vi "Region-det-diagnostics.vi"() -> ()   [LabVIEW 2016]
panel:
  out "Region 3":dbl
  out "millisec gen Q mat":u32
  out "millisec det reg":u32
  out "Region 2":dbl
  out "Region":dbl
  in  "State":dbl[](array[numeric])
  out "Q Matrices":dbl[][][][](array[numeric])
  # "Just for diagnostics (to record the amount of time it takes to load a JSON file as compared with the amount of time to determine the region"
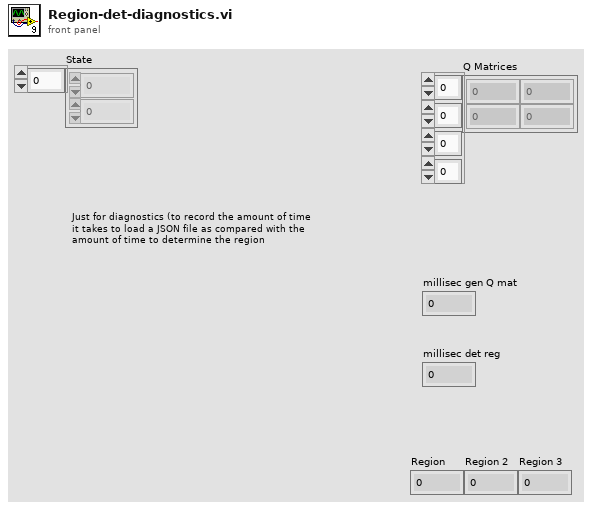
[diagram p1: front panel]
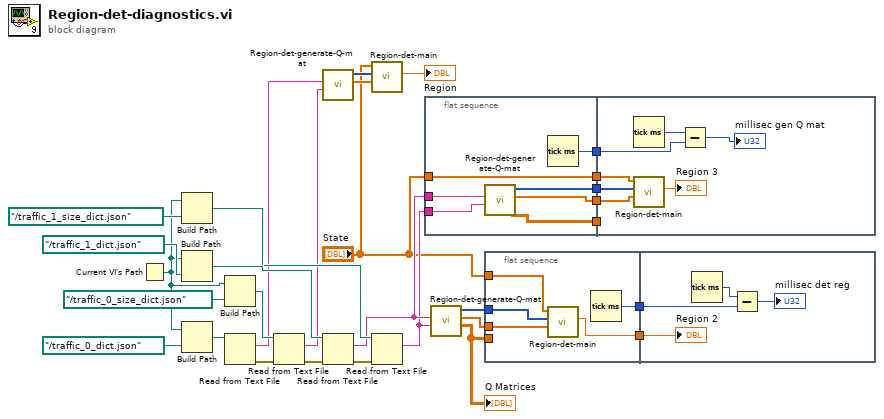
[diagram p0: block diagram]
diagram:
  n1 = Current VI's Path() -> (path=w22:path)
  n2 = Build Path(base path=w22, name or relative path=path "../traffic_1_size_dict.json") -> (appended path=w23:path)
  n3 = Build Path(base path=w22, name or relative path=path "../traffic_1_dict.json") -> (appended path=w26:path)
  n4 = Build Path(base path=w22, name or relative path=path "../traffic_0_dict.json") -> (appended path=w30:path)
  n5 = Build Path(base path=w22, name or relative path=path "../traffic_0_size_dict.json") -> (appended path=w27:path)
  n6 = Read from Text File(file (use dialog)=w30) -> (text=w18:string, error out=w21:errorcluster)  [unwired: 3 in, 2 out]
  n7 = Read from Text File(file (use dialog)=w27, error in=w21) -> (text=w17:string, error out=w20:errorcluster)  [unwired: 2 in, 2 out]
  n8 = call "Region-det-generate-Q-mat.vi"("Q region size JSON string"=w17, "Q matrix JSON string"=w18) -> ("Index array"=w14:dbl[], "Regions"=w16:i32[])  [unwired: 6 in, 2 out]
  n9 = Read from Text File(file (use dialog)=w26, error in=w20) -> (text=w7:string, error out=w19:errorcluster)  [unwired: 2 in, 2 out]
  n10 = call "Region-det-main.vi"("Index Array"=w14, "Regions"=w16, "State"="State") -> ("Region"=→"Region":dbl)  [unwired: 8 in]
  n11 = Read from Text File(file (use dialog)=w23, error in=w19) -> (text=w6:string)  [unwired: 2 in, 3 out]
  n12 = flat-sequence {
    tunnel: [w37] -> w8
    tunnel: w7 -> [w36]
    tunnel: w6 -> [w35]
    tunnel: [w34] -> w5
    tunnel: "State" -> [w33]
    tunnel: [w33] -> w3
    tunnel: [w32] -> w2
    tunnel: [w31] -> w1
    tunnel: w8 -> [w43]
    tunnel: w5 -> [_]
    tunnel: w3 -> [w41]
    tunnel: w2 -> [w40]
    tunnel: w1 -> [w39]
    frame #0 {
      n13 = call "Region-det-generate-Q-mat.vi"("Q region size JSON string"=w35, "Q matrix JSON string"=w36) -> ("Q Matrices"=w34:dbl[][][][], "Index array"=w32:dbl[], "Regions"=w31:i32[])  [unwired: 6 in, 1 out]
      n14 = Tick Count (ms)() -> (millisecond timer value=w37:u32)
    }
    frame #1 {
      n15 = Tick Count (ms)() -> (millisecond timer value=w44:u32)
      n16 = call "Region-det-main.vi"("Index Array"=w40, "Regions"=w39, "State"=w41) -> ("Region"=→"Region 3":dbl)  [unwired: 8 in]
      n17 = Subtract(x=w44, y=w43) -> (x-y=→"millisec gen Q mat":u32)
    }
  }
  n18 = call "Region-det-generate-Q-mat.vi"("Q region size JSON string"=w6, "Q matrix JSON string"=w7) -> ("Q Matrices"=w12:dbl[][][][], "Index array"=w13:dbl[], "Regions"=w11:i32[])  [unwired: 6 in, 1 out]
  "Q Matrices" <- w12
  n19 = flat-sequence {
    tunnel: "State" -> [w49]
    tunnel: w13 -> [w47]
    tunnel: w12 -> [_]
    tunnel: w11 -> [w48]
    tunnel: [w46] -> w10
    tunnel: [w45] -> w9
    tunnel: w10 -> [w53]
    tunnel: w9 -> [w51]
    frame #0 {
      n20 = call "Region-det-main.vi"("Index Array"=w47, "Regions"=w48, "State"=w49) -> ("Region"=w46:dbl)  [unwired: 8 in]
      n21 = Tick Count (ms)() -> (millisecond timer value=w45:u32)
    }
    frame #1 {
      n22 = Tick Count (ms)() -> (millisecond timer value=w52:u32)
      n23 = Subtract(x=w52, y=w51) -> (x-y=→"millisec det reg":u32)
      "Region 2" <- w53
    }
  }
